vi "Process_Setting_UI.vi"(10 "ProcessSettingIn":T12[](array[typedef]), 11 "Vision_Image_In":T1(plugin-control)) -> (1 "Cancel?":bool, 2 "ProcessSettingOut":T12[](array[typedef]))   [LabVIEW 2019]
uses:
  <vilib>/vision/driver/NI_Vision_Acquisition_Software.lvlib
  <vilib>/userdefined/High Color/IMAQdx.ctl
  Controls/Process_UIAction.ctl
  Controls/UI_Process_Type.ctl
  Controls/ProcessDataEntry_Action.ctl
  Controls/Control_EnDisable_Action.ctl
  Controls/BinaryMonoParam_Type.ctl
  Controls/OperatorsParam_Type.ctl
  Controls/FiltersParam_Type.ctl
  Controls/GrayMorphologyParam_Type.ctl
  Controls/LookupTableParam.ctl
  Controls/ParticleFilterParam_Type.ctl
  Controls/MaskParam_Type.ctl
  Controls/MaskROIList_Action.ctl
  Controls/Process_Type.ctl
  <vilib>/vision/Image Controls.llb/IMAQ Image.ctl
  Controls/Process_Setting.ctl
  Controls/ExtractPlanParam_Type.ctl
  Ctrl/VisionProcessName.ctl
panel:
  out "offset past match":i32
  in  "Save":bool
  out "Vision_Image_Show":T1(plugin-control)
  in  "Tab":T2=enum."ExtractPlane"
  in  "ExtractPlanParam":T3={"Color Plane"=enum."Green"}
  in  "BinaryMonoParam":T4={"Look For"=enum."Bright Objects", "Threshold"={120.0, 255.0}} {"Threshold" scale=0.0..255.0}
  in  "OperatorsParam":T5
  out "Operators_Image":T1(plugin-control)
  in  "GrayMorphologyParam":T6={"Operation"=enum."AutoM", "Structuring Element"=[[1, 1, 1], [1, 1, 1], [1, 1, 1]], "Square/Hexa (Square)"=FALSE, "Number of iterations"=1}
  in  "FiltersParam":T7={"Kernel"=[[1.0, 1.0, 1.0], [1.0, 1.0, 1.0], [1.0, 1.0, 1.0]], "Kernel Size"=0, "Filter Size X"=0, "Filter Size Y"=0, "Tolerance %"=0, "Divider"=0.0, "FilterFunction"=enum."Smoothing - Low Pass", "Sigma"=0.0, "LThres"=0.0, "HThresh"=0.0, "Windows Size"=0} {"Kernel Size" min=3 max=7 step=2}
  in  "LookupTableParam":T8={"Function"=enum."Power X", "Power Value"=1.5}
  in  "ParticleFilterParam":T9={"Selection Values"=[], "Keep/Remove Particles (F)"=FALSE, "Reject Border? (F)"=FALSE, "Fill Holes? (F)"=FALSE, "Connectivity 4/8 (8)"=TRUE} {"Selection Values"."Measurement Parameter" items=["Center of Mass X", "Center of Mass Y", "First Pixel X", "First Pixel Y", "Bounding Rect Left", "Bounding Rect Top", "Bounding Rect Right", "Bounding Rect Bottom", "Max Feret Diameter Start X", "Max Feret Diameter Start Y", "Max Feret Diameter End X", "Max Feret Diameter End Y", "Max Horiz. Segment Length Left", "Max Horiz. Segment Length Right", "Max Horiz. Segment Length Row", "-", "Bounding Rect Width", "Bounding Rect Height", "Bounding Rect Diagonal", "Perimeter", "Convex Hull Perimeter", "Holes' Perimeter", "Max Feret Diameter", "Equivalent Ellipse Major Axis", "Equivalent Ellipse Minor Axis", "Equivalent Ellipse Minor Axis (Feret)", "Equivalent Rect Long Side", "Equivalent Rect Short Side", "Equivalent Rect Diagonal", "Equivalent Rect Short Side (Feret)", "Average Horiz. Segment Length", "Average Vert. Segment Length", "Hydraulic Radius", "Waddel Disk Diameter", "-", "Area", "Holes' Area", "Particle & Holes' Area", "Convex Hull Area", "Image Area", "-", "Number of Holes", "Number of Horiz. Segments", "Number of Vert. Segments", "-", "Orientation", "Max Feret Diameter Orientation", "-", "% Area/Image Area", "% Area/(Particle & Holes' Area)", "Ratio of Equivalent Ellipse Axes", "Ratio of Equivalent Rect Sides", "-", "Elongation Factor", "Compactness Factor", "Heywood Circularity Factor", "Type Factor", "-", "Sum X", "Sum Y", "Sum XX", "Sum XY", "Sum YY", "Sum XXX", "Sum XXY", "Sum XYY", "Sum YYY", "-", "Moment of Inertia XX", "Moment of Inertia XY", "Moment of Inertia YY", "Moment of Inertia XXX", "Moment of Inertia XXY", "Moment of Inertia XYY", "Moment of Inertia YYY", "Norm. Moment of Inertia XX", "Norm. Moment of Inertia XY", "Norm. Moment of Inertia YY", "Norm. Moment of Inertia XXX", "Norm. Moment of Inertia XXY", "Norm. Moment of Inertia XYY", "Norm. Moment of Inertia YYY", "Hu Moment 1", "Hu Moment 2", "Hu Moment 3", "Hu Moment 4", "Hu Moment 5", "Hu Moment 6", "Hu Moment 7"]; "Selection Values"."Range Lower Value" format="%.2f"; "Selection Values"."Range Upper Value" format="%.2f"}
  in  "MaskParam":T11
  in  "Remove":bool
  in  "Add":bool
  in  "Process Steps":i32(listbox)
  in  "Cancel":bool
  in  "Done":bool
  # "Minimum"
  # "Maximum"
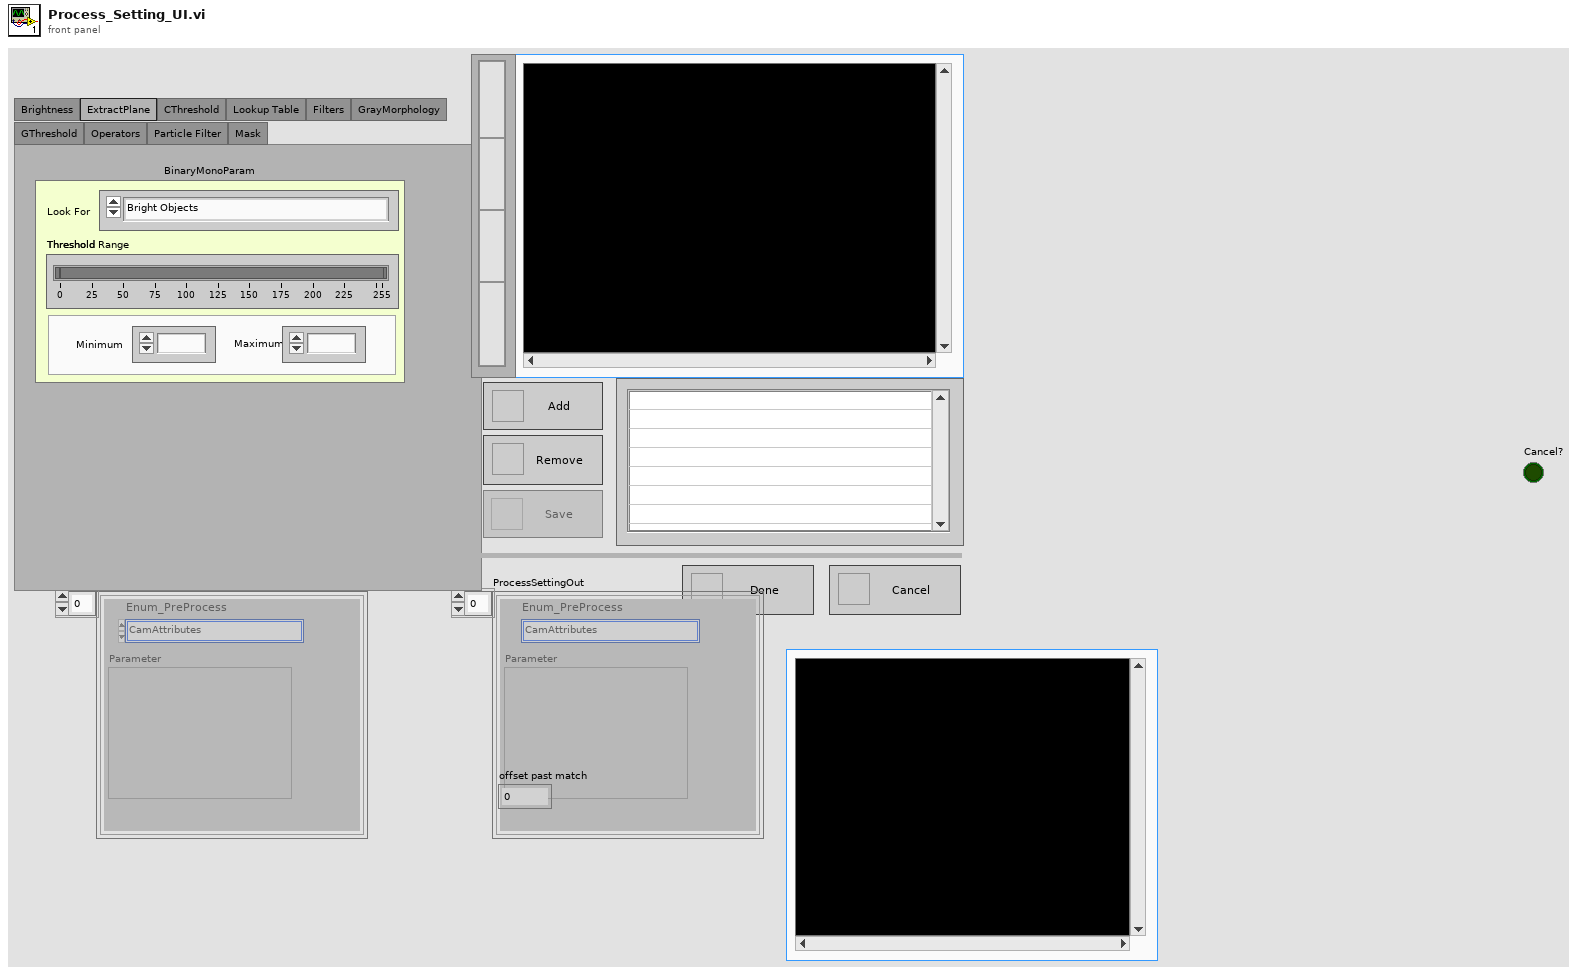
[diagram p1: front panel]
types:
  T1 = typedef "IMAQ Image.ctl" = refnum<image>
  T2 = typedef "UI_Process_Type.ctl" = enum32{"None", "Brightness", "ExtractPlane", "CThreshold", "Lookup Table", "Filters", "GrayMorphology", "GThreshold", "Operators", "Particle Filter", "Mask"}
  T3 = typedef "ExtractPlanParam_Type.ctl" = cluster{"Color Plane":enum16{"Red", "Green", "Blue", "Hue", "Saturation", "Luminance", "Value", "Intensity"}}
  T4 = typedef "BinaryMonoParam_Type.ctl" = cluster{"Look For":enum16{"Bright Objects", "Dark Objects", "Gray Objects"}, "Threshold":cluster{dbl, dbl}}
  T5 = typedef "OperatorsParam_Type.ctl" = cluster{"Actions":enum16{"Add", "Subtract", "Multiply", "Divide", "Multiply Divide", "Modulo", "Absolutio Difference", "---------------------------------", "And", "Not And", "Or", "Not Or", "Exclusive Or", "Not Exclusive Or", "Logical Difference", "----------------------------------", "Mask"}, "Select Mode:":enum32{"Constant", "Image"}, "Color Box":u32, "Image Path":path}
  T6 = typedef "GrayMorphologyParam_Type.ctl" = cluster{"Operation":enum32{"AutoM", "Close", "Dilate", "Erode", "Gradient", "Gradient in", "Gradient out", "HitMiss", "Open", "PClose", "POpen", "Thick", "Thin"}, "Structuring Element":i32[][], "Square/Hexa (Square)":bool, "Number of iterations":i32}
  T7 = typedef "FiltersParam_Type.ctl" = cluster{"Kernel":sgl[][], "Kernel Size":i32, "Filter Size X":i32, "Filter Size Y":i32, "Tolerance %":i32, "Divider":sgl, "FilterFunction":enum16{"Smoothing - Low Pass", "Smoothing - Local Average", "Smoothing - Guassian", "Smoothing - Median", "------------------------------------", "Edge Detection - Laplacian", "Edge Detection - Diff", "Edge Detection - Prewitt", "Edge Detection - Sobel", "Edge Detection - Roberts", "Edge Detection - Canny", "Edge Detection - Gradient", "Edge Detection - Sigma", "----------------------------------------", "Convolution - Highlight Details", "Convolution - Custom"}, "Sigma":sgl, "LThres":sgl, "HThresh":sgl, "Windows Size":i32}
  T8 = typedef "LookupTableParam.ctl" = cluster{"Function":enum16{"Equalizer", "Reverse", "Logarithmic", "Exponential", "Square", "Square Root", "Power X", "Power 1/X"}, "Power Value":sgl}
  T9 = typedef "ParticleFilterParam_Type.ctl" = cluster{"Selection Values":cluster{"Measurement Parameter":T10, "Range Lower Value":dbl, "Range Upper Value":dbl, "Range":bool, "Measurement Type":bool}[], "Keep/Remove Particles (F)":bool, "Reject Border? (F)":bool, "Fill Holes? (F)":bool, "Connectivity 4/8 (8)":bool}
  T10 = typedef "Particle Parameters" = i32
  T11 = typedef "MaskParam_Type.ctl" = cluster{"Function":enum16{"Inside", "Outside"}, "ROI List":i32, "ROI":cluster{"Global Rectangle":i32[], "Contours":cluster{"Contour Type":u32, "ROI Type":u32, "Points":i32[]}[]}[], "Creat ROI":bool, "Delete ROI":bool, "Enabled/Disabled":bool, "Color Box":u32, "Last Mouse Position":cluster{"X":i32, "Y":i32}}
  T12 = typedef "Process_Setting.ctl" = cluster{"Enum_PreProcess":T13, "Parameter":string}
  T13 = typedef "VisionProcessName.ctl" = enum16{"*CamParameter*", "CamAttributes", "*Preprocess*", "CG_Brightness", "C_Plane Extraction", "C_Threshold", "G_Lookup Table", "G_Threshold"}
  T14 = enum8{"Enabled", "Disabled", "Disabled and Grayed Out"}
  T15 = typedef "ProcessDataEntry_Action.ctl" = enum16{"Intial", "UpdateSteps", "ReallAllSteps", "ReadStep"}
  T16 = typedef "Image Type" = u32
  T17 = typedef "Process_UIAction.ctl" = cluster{"Process_UIActionCmd":enum16{"Init", "SingleStep", "RunAllSteps", "RemoveSteps", "PreTest", "Exist"}, "Process_UIParam":variant, "EventName":string}
  T18 = typedef "IMAQdx.ctl" = refnum<k21>
  T19 = typedef "Control_EnDisable_Action.ctl" = enum16{"Store Ref", "Add Mode", "Select Mode", "Enable All", "OnePageEnable", "OnePageDisable", "AllPageDisable", "AllPageEnable", "PageRefOut"}
  T20 = cluster{"Color Plane":enum16{"Red", "Green", "Blue", "Hue", "Saturation", "Luminance", "Value", "Intensity"}}
  T21 = typedef "MaskROIList_Action.ctl" = enum16{"initialize", "SaveAll", "ReadAll", "Append", "Replace", "DeleteIndex"}
  T22 = typedef "Process_Type.ctl" = enum16{"None", "ExtractPlane", "BinaryMono", "Operators", "GrayMorphology", "Filters", "Lookup Table", "Particle Filter", "Mask"}
  T23 = enum16{"Smoothing - Low Pass", "Smoothing - Local Average", "Smoothing - Guassian", "Smoothing - Median", "------------------------------------", "Edge Detection - Laplacian", "Edge Detection - Diff", "Edge Detection - Prewitt", "Edge Detection - Sobel", "Edge Detection - Roberts", "Edge Detection - Canny", "Edge Detection - Gradient", "Edge Detection - Sigma", "----------------------------------------", "Convolution - Highlight Details", "Convolution - Custom"}
  T24 = enum16{"Bright Objects", "Dark Objects", "Gray Objects"}
  T25 = cluster{"Look For":enum16{"Bright Objects", "Dark Objects", "Gray Objects"}, "Threshold Range Gray":cluster{dbl, dbl}}
  T26 = cluster{"Global Rectangle":i32[], "Contours":cluster{"Contour Type":u32, "ROI Type":u32, "Points":i32[]}[]}
  T27 = cluster{"Contour Type":u32, "ROI Type":u32, "Points":i32[]}[]
  T28 = cluster{"Global Rectangle":i32[], "Contours":cluster{"Contour Type":u32, "ROI Type":u32, "Points":i32[]}[]}[]
  T29 = typedef "UI_Process_Type.ctl" = enum32{"None", "Brightness", "ExtractPlane", "Lookup Table", "Filters", "GrayMorphology", "BinaryMono", "Operators", "Particle Filter", "Mask"}
  T30 = enum16{"Init", "SingleStep", "RunAllSteps", "RemoveSteps", "PreTest", "Exist"}
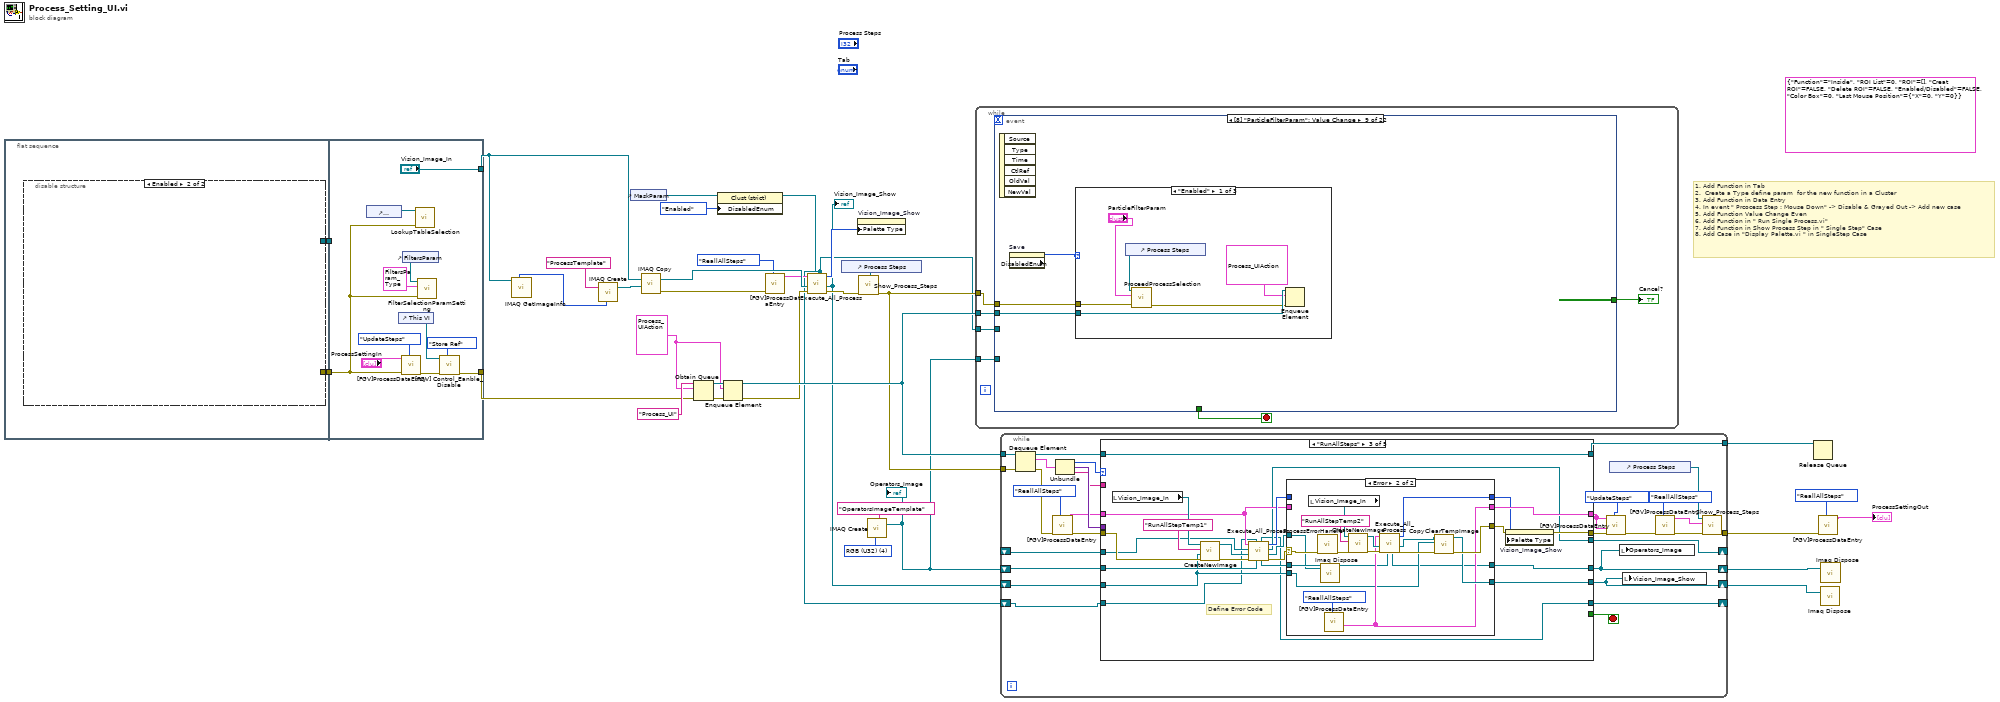
[diagram p0: block diagram]
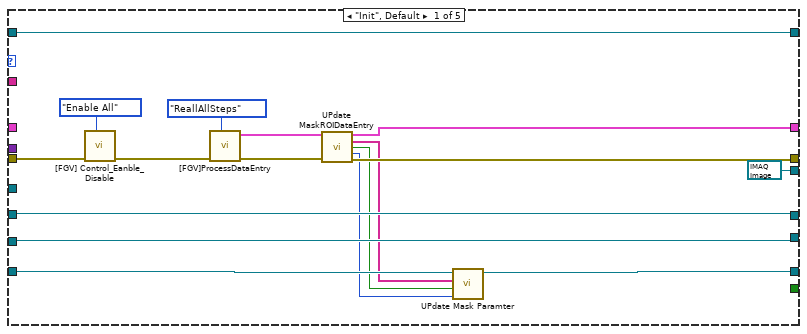
[diagram p2: hidden frame]
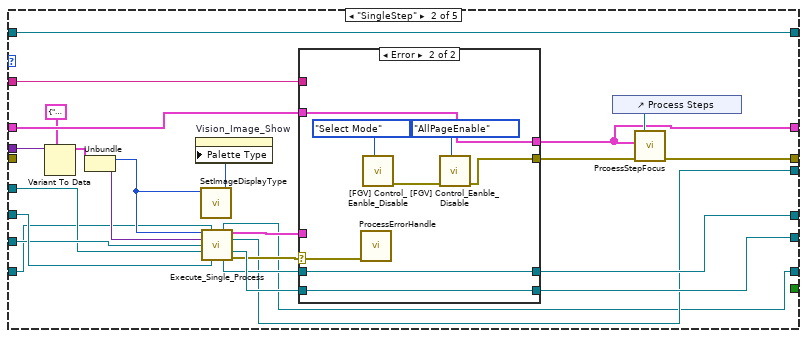
[diagram p3: hidden frame]
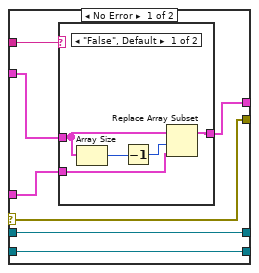
[diagram p4: hidden frame]
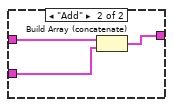
[diagram p5: hidden frame]
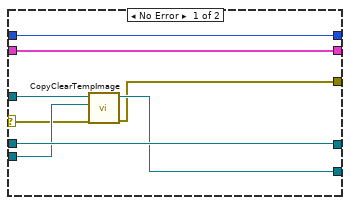
[diagram p6: hidden frame]
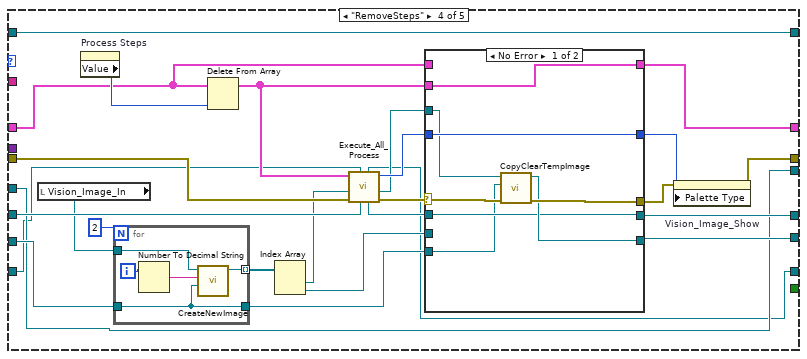
[diagram p7: hidden frame]
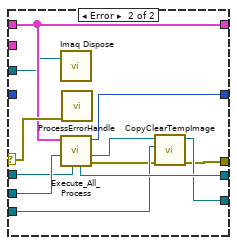
[diagram p8: hidden frame]
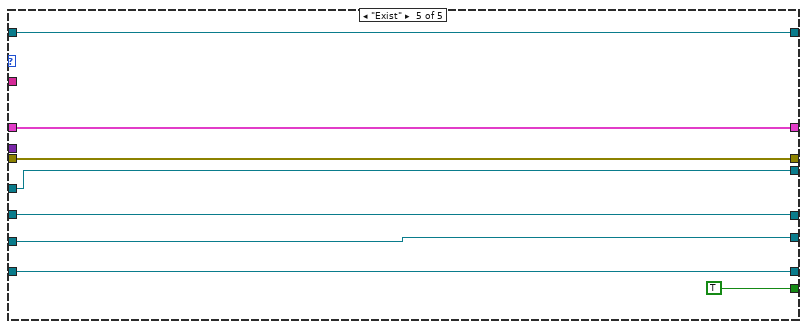
[diagram p9: hidden frame]
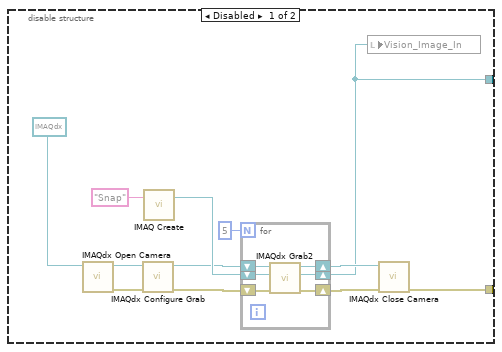
[diagram p10: hidden frame]
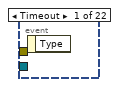
[diagram p11: hidden frame]
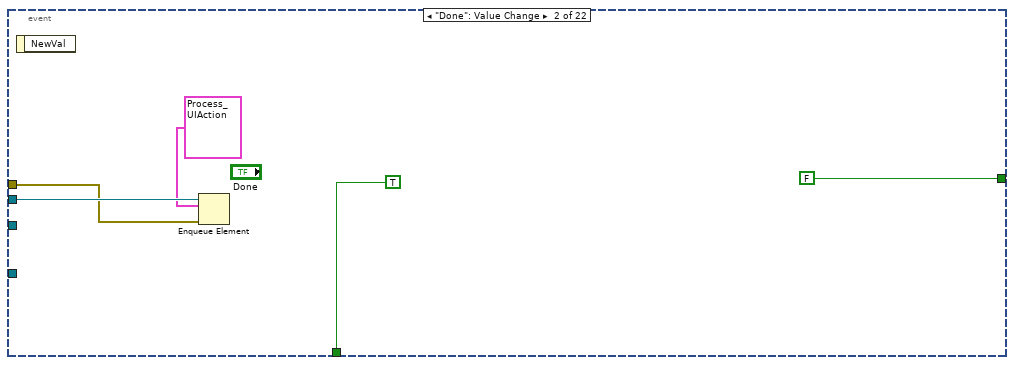
[diagram p12: hidden frame]
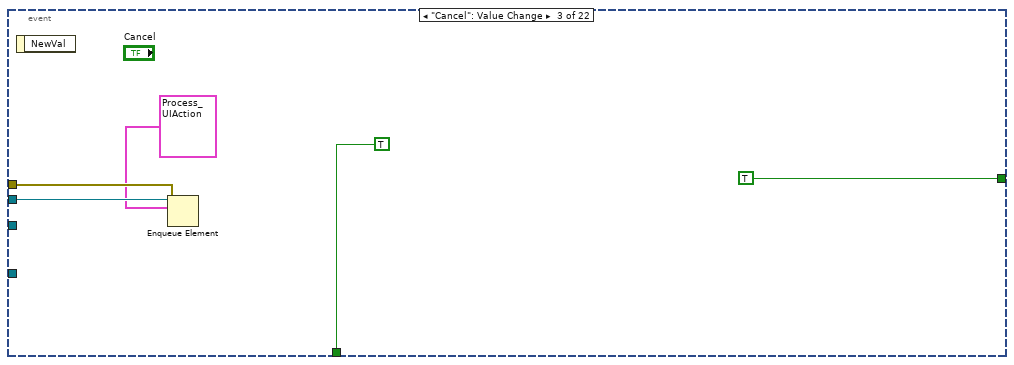
[diagram p13: hidden frame]
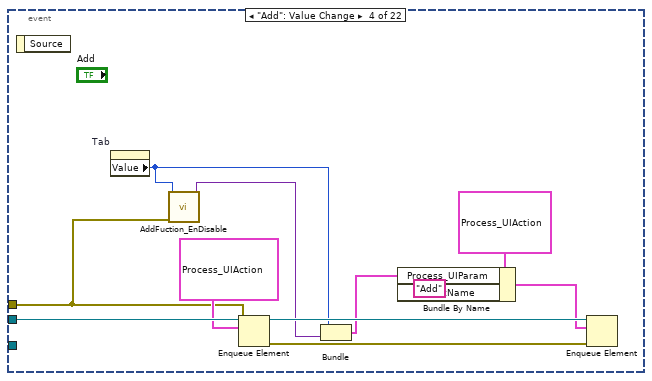
[diagram p14: hidden frame]
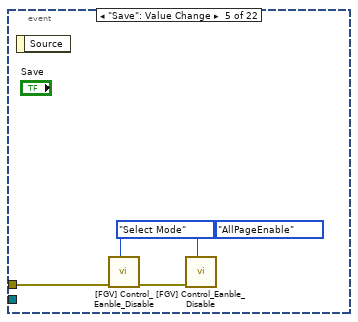
[diagram p15: hidden frame]
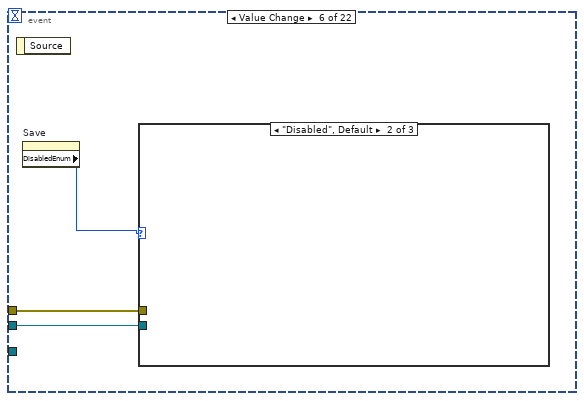
[diagram p16: hidden frame]
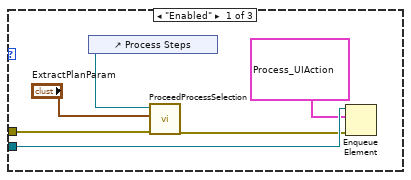
[diagram p17: hidden frame]
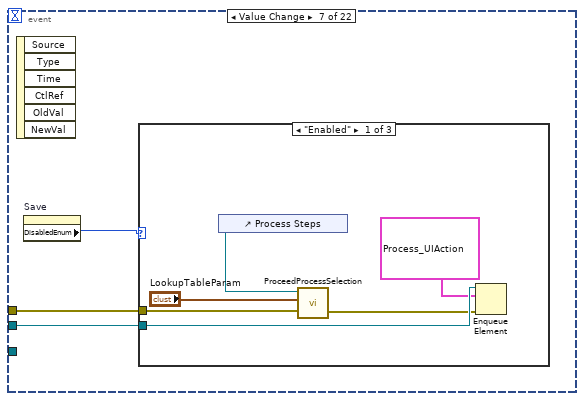
[diagram p19: hidden frame]
diagram:
  (unwired) T11 {"Function"=enum."Inside", "ROI List"=0, "ROI"=[], "Creat ROI"=FALSE, "Delete ROI"=FALSE, "Enabled/Disabled"=FALSE, "Color Box"=0, "Last Mouse Position"={"X"=0, "Y"=0}} ("MaskParam")
  w18 = T16 4 items=["Grayscale (U8)", "Grayscale (I16)", "Grayscale (SGL)", "Complex (CSG)", "RGB (U32)", "HSL (U32)", "RGB (U64)", "Grayscale (U16)"] ("Image Type")
  w21 = T17 {"Process_UIActionCmd"=enum."Init", "Process_UIParam"=variant, "EventName"=""} ("Process_UIAction")
  # "1. Add Function in Tab \n2.  Create a Type define param  for the new function in a Cluster \n3. Add Function in Data Entry\n4. In event \" Prcocess Step : Mouse Down\" -> Disable & Grayed Out -> Add new case \n5. Add Function Value Change Even\n6. Add Function in \" Run Single Process.vi\"\n7. Add Function in Show Process Step in \" Single Step\" Case\n8. Add Case in \"Display Palette.vi \" in SingleStep Case"
  n1 = flat-sequence {
    tunnel: [w37] -> w31
    tunnel: [w36] -> w30
    tunnel: ["Vision_Image_In"] -> w33
    tunnel: [w62] -> w14
    tunnel: w31 -> [w57]
    tunnel: w30 -> [_]
    frame #0 {
      n2 = disable-structure shown="Enabled" {
        disable-tunnel: [w43 _] -> w37
        disable-tunnel: [w38 _] -> w36
        frame Disabled {
          n3 = call <vilib>:"IMAQdx Open Camera.vi"("Session In"=T18 refnum) -> ("error out"=w41:errorcluster, "Session Out"=w48:T18)  [unwired: 2 in, 7 out]
          n4 = call <vilib>:"IMAQdx Configure Grab.vi"("error in"=w41, "Session In"=w48) -> ("error out"=w40:errorcluster, "Session Out"=w42:T18)  [unwired: 8 in]
          n5 = call "IMAQ Create"("Image Name"="Snap") -> ("New Image"=w46:T1)  [unwired: 3 in, 2 out]
          n6 = for {
            N: 5 -> [_]
            shift-right: [w52] -> w38
            shift-left: w46 -> [w53]
            shift-right: [w55] -> w49
            shift-left: w42 -> [w51]
            shift-right: [w54] -> w47
            shift-left: w40 -> [w50]
            n7 = call <vilib>:"IMAQdx Grab2.vi"("error in"=w50, "Image In"=w53, "Session In"=w51) -> ("error out"=w54:errorcluster, "Image Out"=w52:T1, "Session Out"=w55:T18)  [unwired: 5 in, 1 out]
          }
          n8 = local write "Vision_Image_In"(w38) -> ()
          n9 = call <vilib>:"IMAQdx Close Camera.vi"("error in"=w47, "Session In"=w49) -> ("error out"=w43:errorcluster)  [unwired: 9 out]
        }
        frame Enabled {
        }
      }
    }
    frame #1 {
      n10 = control-ref of="LookupTableParam"() -> (w56:refnum<vi>)
      n11 = control-ref of="This VI"() -> (w61:refnum<vi>)
      n12 = call "[FGV]ProcessDataEntry.vi"("ProcessDataEntry_Action"=ProcessDataEntry_Action."UpdateSteps", "Error In"=w57, "AllProcessSetting In"="ProcessSettingIn") -> ("Error Out"=w63:errorcluster)  [unwired: 5 in, 3 out]
      n13 = control-ref of="FiltersParam"() -> (w59:refnum<vi>)
      n14 = call "LookupTableSelection.vi"("Error In"=w57, "LookupTableParam"=w56) -> ()  [unwired: 9 in, 1 out]
      n15 = call "FilterSelectionParamSetting.vi"("Error In"=w57, 10:"FiltersParam"=T7 {"Kernel"=[[1.0, 1.0, 1.0], [1.0, 1.0, 1.0], [1.0, 1.0, 1.0]], "Kernel Size"=0, "Filter Size X"=0, "Filter Size Y"=0, "Tolerance %"=0, "Divider"=0.0, "FilterFunction"=enum."Smoothing - Low Pass", "Sigma"=0.0, "LThres"=0.0, "HThresh"=0.0, "Windows Size"=0} ("FiltersParam"), 11:"FiltersParam"=w59) -> ()  [unwired: 8 in, 1 out]
      n16 = call "[FGV] Control_Eanble_Disable.vi"("Control_EnDisable_Action"=Control_EnDisable_Action."Store Ref", "Error In"=w63, "This VI"=w61) -> ("Error Out"=w62:errorcluster)  [unwired: 7 in, 1 out]
    }
  }
  n17 = call "IMAQ GetImageInfo"("Image"=w33) -> ("Image Type"=w19:T16)  [unwired: 3 in, 7 out]
  n18 = call "IMAQ Create"("Image Name"="ProcessTemplate", "Image Type"=w19) -> ("New Image"=w34:T1)  [unwired: 3 in, 1 out]
  n19 = control-ref of="MaskParam"() -> (w4:refnum<vi>)
  n20 = call "IMAQ Copy"("Image Dst"=w34, "Image Src"=w33) -> ("error out"=w10:errorcluster, "Image Dst Out"=w29:T1)  [unwired: 4 in]
  n21 = Obtain Queue(name (unnamed)="Process_UI", element data type=w21, error in (no error)=w14) -> (queue out=w26:refnum<queue>, error out=w22:errorcluster)  [unwired: 2 in, 1 out]
  n22 = property class="Clust (strict)"(reference=w4, "DisabledEnum"=T14."Enabled" ("Disabled")) -> (reference out=w2:refnum<vi>)  [unwired: 1 in, 1 out]
  n23 = Enqueue Element(queue=w26, element=w21, error in (no error)=w22) -> (queue out=w23:refnum<queue>, error out=w5:errorcluster)  [unwired: 1 in, 1 out]
  n24 = call "[FGV]ProcessDataEntry.vi"("ProcessDataEntry_Action"=ProcessDataEntry_Action."ReallAllSteps", "Error In"=w10) -> ("AllProcessSettingOut"=w9:T12[])  [unwired: 6 in, 3 out]
  n25 = call "Execute_All_Process.vi"("MaskParam 2"=w2, "error in (no error)"=w5, "ImageIn"=w29, "ProcessSettingIn"=w9) -> ("error out"=w16:errorcluster, "Image Out"=w15:T1, "Palette Type"=w28:u32, "MaskParam 3"=w3:refnum<vi>)  [unwired: 2 in, 2 out]
  "Vision_Image_Show" <- w15
  n26 = control-ref of="Process Steps"() -> (w32:refnum<vi>)
  n27 = property on="Vision_Image_Show" class="ImageControl"("Palette Type"=w28) -> ()  [unwired: 2 in, 2 out]
  n28 = call "Show_Process_Steps.vi"("error in (no error)"=w16, "ProcessSteps"=w32) -> ("error out"=w17:errorcluster)  [unwired: 9 in]
  n29 = call "IMAQ Create"("Image Name"="OperatorsImageTemplate", "Image Type"=w18) -> ("New Image"=w12:T1)  [unwired: 3 in, 1 out]
  "Operators_Image" <- w12
  n30 = while {
    tunnel: w17 -> [w70]
    tunnel: w23 -> [w71]
    tunnel: w12 -> [w69]
    tunnel: w3 -> [w67]
    stop <- w72 stop-if-true
    n31 = event shown="[8] \"ParticleFilterParam\": Value Change" {
      selector: _ -> [_ _ _ _ _ _ _ _ _ _ _ _ _ _ _ _ _ _ _ _ _ _]
      dyn-events: _ -> [_ _ _ _ _ _ _ _ _ _ _ _ _ _ _ _ _ _ _ _ _ _]
      timeout: _ -> [_ _ _ _ _ _ _ _ _ _ _ _ _ _ _ _ _ _ _ _ _ _]
      tunnel: [_ TRUE TRUE _ _ _ _ _ _ _ _ _ _ _ _ _ _ _ _ _ _ _] -> w72
      tunnel: w71 -> [_ w76 w81 w93 _ w100 w109 w118 w127 w143 _ _ w170 w189 _ w232 w237 w274 w310 w322 w348 w385]
      tunnel: w70 -> [_ w75 w80 w87 w94 w98 w107 w116 w125 w142 w149 w150 w171 w183 _ w231 w236 _ w311 w320 w349 _]
      tunnel: w69 -> [_ _ _ _ _ _ _ _ _ _ _ _ w169 _ _ _ _ _ _ _ w346 _]
      tunnel: [_ FALSE ("Cancel?") TRUE ("Cancel?") _ _ _ _ _ _ _ _ _ _ _ _ _ _ _ _ _ _ _] -> w68
      tunnel: w67 -> [_ _ _ _ _ _ _ _ _ _ _ _ _ _ _ _ w234 w272 w312 w321 w347 w378]
      event Timeout {
        n32 = event-data() -> ()  [unwired: 1 in, 1 out]
      }
      event "Done": Value Change {
        n33 = event-data() -> ()  [unwired: 1 in, 1 out]
        n34 = Enqueue Element(queue=w76, element=T17 {"Process_UIActionCmd"=enum."Exist", "Process_UIParam"=variant, "EventName"=""}, error in (no error)=w75) -> ()  [unwired: 1 in, 3 out]
      }
      event "Cancel": Value Change {
        n35 = event-data() -> ()  [unwired: 1 in, 1 out]
        n36 = Enqueue Element(queue=w81, element=T17 {"Process_UIActionCmd"=enum."Exist", "Process_UIParam"=variant, "EventName"=""}, error in (no error)=w80) -> ()  [unwired: 1 in, 3 out]
      }
      event "Add": Value Change {
        n37 = event-data() -> ()  [unwired: 1 in, 1 out]
        n38 = property on="Tab" class="TabCtl (strict)"() -> ("Value"=w86:T2)  [unwired: 2 in, 2 out]
        n39 = call "AddFuction_EnDisable.vi"("error in (no error)"=w87, "Value"=w86) -> ("Selected Param"=w84:variant)  [unwired: 9 in]
        n40 = Enqueue Element(queue=w93, element=T17 {"Process_UIActionCmd"=enum."RunAllSteps", "Process_UIParam"=variant, "EventName"=""}, error in (no error)=w87) -> (queue out=w91:refnum<queue>, error out=w83:errorcluster)  [unwired: 1 in, 1 out]
        n41 = Bundle("Value"=w86, "Selected Param"=w84) -> (w89:cluster{"Value":T2, "Selected Param":variant})  [unwired: 1 in]
        n42 = Bundle By Name(cluster=T17 {"Process_UIActionCmd"=enum."SingleStep", "Process_UIParam"=variant, "EventName"=""} ("element"), "Process_UIParam"=w89, "EventName"="Add") -> (w88:T17)
        n43 = Enqueue Element(queue=w91, element=w88, error in (no error)=w83) -> ()  [unwired: 1 in, 3 out]
      }
      event "Save": Value Change {
        n44 = event-data() -> ()  [unwired: 1 in, 1 out]
        n45 = call "[FGV] Control_Eanble_Disable.vi"("Control_EnDisable_Action"=Control_EnDisable_Action."Select Mode", "Error In"=w94) -> ("Error Out"=w96:errorcluster)  [unwired: 8 in, 1 out]
        n46 = call "[FGV] Control_Eanble_Disable.vi"("Control_EnDisable_Action"=Control_EnDisable_Action."AllPageEnable", "Error In"=w96) -> ()  [unwired: 8 in, 2 out]
      }
      event Value Change {
        n47 = event-data() -> ()  [unwired: 1 in, 1 out]
        n48 = property on="Save" class="Bool"() -> ("DisabledEnum"=w99:T14)  [unwired: 2 in, 2 out]
        n49 = case shown="\"Disabled\", Default" w99 {
          tunnel: w100 -> [w106 _ _]
          tunnel: w98 -> [w101 _ _]
          frame "Enabled" {
            n50 = control-ref of="Process Steps"() -> (w103:refnum<vi>)
            n51 = call "ProceedProcessSelection.vi"("Error In"=w101, "Selected Param"="ExtractPlanParam", "MulticolumnListbox in"=w103) -> ("error out"=w104:errorcluster)  [unwired: 8 in]
            n52 = Enqueue Element(queue=w106, element=T17 {"Process_UIActionCmd"=enum."RunAllSteps", "Process_UIParam"=variant, "EventName"=""}, error in (no error)=w104) -> ()  [unwired: 1 in, 3 out]
          }
          frame "Disabled", Default {
          }
          frame "Disabled and Grayed Out" {
          }
        }
      }
      event Value Change {
        n53 = event-data() -> ()  [unwired: 1 in, 6 out]
        n54 = property on="Save" class="Bool"() -> ("DisabledEnum"=w108:T14)  [unwired: 2 in, 2 out]
        n55 = case shown="\"Enabled\"" w108 {
          tunnel: w109 -> [w115 _ _]
          tunnel: w107 -> [w111 _ _]
          frame "Enabled" {
            n56 = control-ref of="Process Steps"() -> (w112:refnum<vi>)
            n57 = call "ProceedProcessSelection.vi"("Error In"=w111, "Selected Param"="LookupTableParam", "MulticolumnListbox in"=w112) -> ("error out"=w113:errorcluster)  [unwired: 8 in]
            n58 = Enqueue Element(queue=w115, element=T17 {"Process_UIActionCmd"=enum."RunAllSteps", "Process_UIParam"=variant, "EventName"=""}, error in (no error)=w113) -> ()  [unwired: 1 in, 3 out]
          }
          frame "Disabled", Default {
          }
          frame "Disabled and Grayed Out" {
          }
        }
      }
      event Value Change {
        n59 = event-data() -> ()  [unwired: 1 in, 1 out]
        n60 = property on="Save" class="Bool"() -> ("DisabledEnum"=w117:T14)  [unwired: 2 in, 2 out]
        n61 = case shown="\"Enabled\"" w117 {
          tunnel: w118 -> [w124 _ _]
          tunnel: w116 -> [w120 _ _]
          frame "Enabled" {
            n62 = control-ref of="Process Steps"() -> (w121:refnum<vi>)
            n63 = call "ProceedProcessSelection.vi"("Error In"=w120, "Selected Param"="GrayMorphologyParam", "MulticolumnListbox in"=w121) -> ("error out"=w122:errorcluster)  [unwired: 8 in]
            n64 = Enqueue Element(queue=w124, element=T17 {"Process_UIActionCmd"=enum."RunAllSteps", "Process_UIParam"=variant, "EventName"=""}, error in (no error)=w122) -> ()  [unwired: 1 in, 3 out]
          }
          frame "Disabled", Default {
          }
          frame "Disabled and Grayed Out" {
          }
        }
      }
      event Value Change {
        n65 = event-data() -> ()  [unwired: 1 in, 6 out]
        n66 = property on="Save" class="Bool"() -> ("DisabledEnum"=w126:T14)  [unwired: 2 in, 2 out]
        n67 = case shown="\"Enabled\"" w126 {
          tunnel: w127 -> [w133 _ _]
          tunnel: w125 -> [w129 _ _]
          frame "Enabled" {
            n68 = control-ref of="Process Steps"() -> (w130:refnum<vi>)
            n69 = call "ProceedProcessSelection.vi"("Error In"=w129, "Selected Param"="ParticleFilterParam", "MulticolumnListbox in"=w130) -> ("error out"=w131:errorcluster)  [unwired: 8 in]
            n70 = Enqueue Element(queue=w133, element=T17 {"Process_UIActionCmd"=enum."RunAllSteps", "Process_UIParam"=variant, "EventName"=""}, error in (no error)=w131) -> ()  [unwired: 1 in, 3 out]
          }
          frame "Disabled", Default {
          }
          frame "Disabled and Grayed Out" {
          }
        }
      }
      event Value Change {
        n71 = event-data() -> ()  [unwired: 1 in, 6 out]
        n72 = property on="Save" class="Bool" props=["DisabledEnum"]() -> ()  [unwired: 2 in, 3 out]
        n73 = control-ref of="FiltersParam"() -> (w136:refnum<vi>)
        n74 = call "FilterSelectionParamSetting.vi"("Error In"=w142, 10:"FiltersParam"="FiltersParam", 11:"FiltersParam"=w136) -> ("Error Out"=w137:errorcluster)  [unwired: 8 in]
        n75 = call "FilterParamInitial.vi"("Error In"=w137, "FiltersParam"=w136) -> ("Error Out"=w138:errorcluster, "FiltersParam Out"=w134:T7)  [unwired: 8 in]
        n76 = control-ref of="Process Steps"() -> (w140:refnum<vi>)
        n77 = call "ProceedProcessSelection.vi"("Error In"=w138, "Selected Param"=w134, "MulticolumnListbox in"=w140) -> ("error out"=w139:errorcluster)  [unwired: 8 in]
        n78 = Enqueue Element(queue=w143, element=T17 {"Process_UIActionCmd"=enum."RunAllSteps", "Process_UIParam"=variant, "EventName"=""}, error in (no error)=w139) -> ()  [unwired: 1 in, 3 out]
      }
      event Value Change {
        w147 = T7 {"Kernel"=[[1.0, 1.0, 1.0], [1.0, 1.0, 1.0], [1.0, 1.0, 1.0]], "Kernel Size"=3, "Filter Size X"=0, "Filter Size Y"=0, "Tolerance %"=0, "Divider"=0.0, "FilterFunction"=enum."Smoothing - Low Pass", "Sigma"=0.0, "LThres"=0.0, "HThresh"=0.0, "Windows Size"=0}  # FiltersParam
        n79 = event-data() -> ("NewVal"=w146:T23)  [unwired: 1 in, 5 out]
        n80 = control-ref of="FiltersParam"() -> (w144:refnum<vi>)
        n81 = Bundle By Name(cluster=w147, "FilterFunction"=w146) -> (w145:T7)
        n82 = call "FilterParamInitial.vi"("Error In"=w149, "FiltersParam"=w144) -> ("Error Out"=w148:errorcluster)  [unwired: 8 in, 1 out]
        n83 = call "FilterSelectionParamSetting.vi"("Error In"=w148, 10:"FiltersParam"=w145, 11:"FiltersParam"=w144) -> ()  [unwired: 8 in, 1 out]
      }
      event Value Change {
        n84 = event-data() -> ()  [unwired: 1 in, 6 out]
        n85 = control-ref of="LookupTableParam"() -> (w151:refnum<vi>)
        n86 = call "LookupTableSelection.vi"("Error In"=w150, "LookupTableParam"=w151) -> ()  [unwired: 9 in, 1 out]
      }
      event Value Change {
        w154 = 3 ("y")
        n87 = event-data() -> ("NewVal.Select Mode:"=w164:enum32{"Constant", "Image"}, "NewVal.Image Path"=w157:path)  [unwired: 1 in]
        n88 = Path To String(path=w157) -> (string=w156:string)
        n89 = String Length(string=w156) -> (length=w155:i32)
        n90 = Subtract(x=w155, y=w154) -> (x-y=w152:i32)
        n91 = String Subset(string=w156, offset (0)=w152, length (rest)=w154) -> (substring=w153:string)
        n92 = Equal?(x=enum32{"Constant", "Image"}."Image", y=w164) -> (x = y?=w162:bool)
        n93 = Not Equal?(x=w157, y=path "") -> (x != y?=w160:bool)
        n94 = Search 1D Array(1D array=string[] ["png", "jpg", "bmp"], element=w153) -> (index of element=w166:i32)  [unwired: 1 in]
        n95 = Equal?(x=-1, y=w166) -> (x = y?=w159:bool)
        n96 = Compound Arithmetic op=AND(w162, w160, w159) -> (w158:bool)
        n97 = property on="Save" class="Bool"() -> ("DisabledEnum"=w168:T14)  [unwired: 2 in, 2 out]
        n98 = case shown="True" w158 {
          frame False {
          }
          frame True {
            n99 = One Button Dialog(message="Input File Type Error", button name ("OK")="OK") -> ()  [unwired: 1 out]
            n100 = property on="Image Path" class="Path"("Value"=path "") -> ()  [unwired: 2 in, 2 out]
          }
        }
        n101 = case shown="\"Enabled\"" w168 {
          tunnel: w171 -> [w178 _ _]
          tunnel: w170 -> [w176 _ _]
          tunnel: w169 -> [_ _ _]
          frame "Enabled" {
            n102 = control-ref of="Process Steps"() -> (w180:refnum<vi>)
            n103 = call "ProceedProcessSelection.vi"("Error In"=w178, "Selected Param"="OperatorsParam", "MulticolumnListbox in"=w180) -> ("error out"=w177:errorcluster)  [unwired: 8 in]
            n104 = Enqueue Element(queue=w176, element=T17 {"Process_UIActionCmd"=enum."RunAllSteps", "Process_UIParam"=variant, "EventName"=""}, error in (no error)=w177) -> ()  [unwired: 1 in, 3 out]
          }
          frame "Disabled", Default {
          }
          frame "Disabled and Grayed Out" {
          }
        }
      }
      event Mouse Up {
        n105 = event-data() -> ()  [unwired: 1 in, 1 out]
        n106 = control-ref of="BinaryMonoParam"() -> (w185:refnum<vi>)
        n107 = Unbundle("BinaryMonoParam") -> ("Look For"=w186:T24, "Threshold"=w187:cluster{dbl, dbl})
        n108 = property on="Save" class="Bool"() -> ("DisabledEnum"=w188:T14)  [unwired: 2 in, 2 out]
        n109 = call "BinaryMono_SliderControl.vi"("NewVal"="BinaryMonoParam", "Error In"=w183, "Look For"=w186, "Threshold Range Gray"=w187, "Cluster in"=w185) -> ("Error Out"=w182:errorcluster, "BinaryMonoParam Out"=w181:T25)  [unwired: 5 in]
        n110 = case shown="\"Enabled\"" w188 {
          tunnel: w189 -> [w195 _ _]
          tunnel: w182 -> [w191 _ _]
          tunnel: w181 -> [w190 _ _]
          frame "Enabled" {
            n111 = control-ref of="Process Steps"() -> (w194:refnum<vi>)
            n112 = call "ProceedProcessSelection.vi"("Error In"=w191, "Selected Param"=w190, "MulticolumnListbox in"=w194) -> ("error out"=w192:errorcluster)  [unwired: 8 in]
            n113 = Enqueue Element(queue=w195, element=T17 {"Process_UIActionCmd"=enum."RunAllSteps", "Process_UIParam"=variant, "EventName"=""}, error in (no error)=w192) -> ()  [unwired: 1 in, 3 out]
          }
          frame "Disabled", Default {
          }
          frame "Disabled and Grayed Out" {
          }
        }
      }
      event "Process Steps": Mouse Down {
        n114 = event-data() -> ("Mods.Double Click"=w197:bool)  [unwired: 1 in]
        n115 = property on="Save" class="Bool"() -> ("DisabledEnum"=w196:T14)  [unwired: 2 in, 2 out]
        n116 = case shown="\"Disabled and Grayed Out\"" w196 {
          tunnel: w197 -> [_ _ w198]
          frame "Enabled" {
          }
          frame "Disabled", Default {
          }
          frame "Disabled and Grayed Out" {
            n117 = case shown="True" w198 {
              frame False {
              }
              frame True {
                n118 = property on="Process Steps" class="MCListbox (strict)"() -> ("Value"=w202:i32)  [unwired: 2 in, 2 out]
                n119 = call "[FGV]ProcessDataEntry.vi"("ProcessDataEntry_Action"=ProcessDataEntry_Action."ReadStep", "Prcocess Step"=w202) -> ("ProcessSetting Out"=w201:T12)  [unwired: 6 in, 3 out]
                n120 = Unbundle By Name(w201) -> ("Process_Type"=w199:T22, "Parameter"=w200:string)
                n121 = case shown="Default" w199 {
                  tunnel: w200 -> [_ w205]
                  tunnel: w199 -> [_ w204]
                  frame "None" {
                  }
                  frame Default {
                    n122 = property on="Tab" class="TabCtl (strict)"("Value"=w204) -> ()  [unwired: 2 in, 2 out]
                    n123 = call "AddFuction_EnDisable.vi"("Value"=w204) -> ()  [unwired: 10 in, 1 out]
                    n124 = case shown="\"BinaryMono\"" w204 {
                      tunnel: w205 -> [_ w206 w211 w214 w217 w220 w223 w226 w229]
                      frame "None", Default {
                      }
                      frame "ExtractPlane" {
                        n125 = Variant To Data(type=T20 {"Color Plane"=enum."Blue"} ("ExtractPlanParam"), Variant=w206) -> (data=w207:T20)  [unwired: 1 in, 1 out]
                        n126 = local write "ExtractPlanParam"(w207) -> ()
                      }
                      frame "BinaryMono" {
                        n127 = Variant To Data(type=T4 {"Look For"=enum."Dark Objects", "Threshold"={0.0, 134.0}} ("BinaryMonoParam"), Variant=w211) -> (data=w209:T4)  [unwired: 1 in, 1 out]
                        n128 = local write "BinaryMonoParam"(w209) -> ()
                      }
                      frame "Operators" {
                        n129 = Variant To Data(type=T5 {"Actions"=enum."Multiply", "Select Mode:"=enum."Image", "Color Box"=9221012, "Image Path"=path "\\\\Mac\\Home/Desktop/ssss.png"} ("OperatorsParam"), Variant=w214) -> (data=w213:T5)  [unwired: 1 in, 1 out]
                        n130 = local write "OperatorsParam"(w213) -> ()
                      }
                      frame "GrayMorphology" {
                        n131 = Variant To Data(type=T6 {"Operation"=enum."AutoM", "Structuring Element"=[[1, 1, 1], [1, 1, 1], [1, 1, 1]], "Square/Hexa (Square)"=FALSE, "Number of iterations"=1} ("GrayMorphologyParam"), Variant=w217) -> (data=w215:T6)  [unwired: 1 in, 1 out]
                        n132 = local write "GrayMorphologyParam"(w215) -> ()
                      }
                      frame "Filters" {
                        n133 = Variant To Data(type=T7 {"Kernel"=[[1.0, 1.0, 1.0], [1.0, 1.0, 1.0], [1.0, 1.0, 1.0]], "Kernel Size"=0, "Filter Size X"=0, "Filter Size Y"=0, "Tolerance %"=0, "Divider"=0.0, "FilterFunction"=enum."Smoothing - Low Pass", "Sigma"=0.0, "LThres"=0.0, "HThresh"=0.0, "Windows Size"=0} ("FiltersParam"), Variant=w220) -> (data=w218:T7)  [unwired: 1 in, 1 out]
                        n134 = local write "FiltersParam"(w218) -> ()
                      }
                      frame "Lookup Table" {
                        n135 = Variant To Data(type=T8 {"Function"=enum."Equalizer", "Power Value"=0.0} ("LookupTableParam"), Variant=w223) -> (data=w221:T8)  [unwired: 1 in, 1 out]
                        n136 = local write "LookupTableParam"(w221) -> ()
                      }
                      frame "Particle Filter" {
                        n137 = Variant To Data(type=T9 {"Selection Values"=[{"Measurement Parameter"=0, "Range Lower Value"=0.0, "Range Upper Value"=0.0, "Range"=FALSE, "Measurement Type"=FALSE}], "Keep/Remove Particles (F)"=FALSE, "Reject Border? (F)"=FALSE, "Fill Holes? (F)"=FALSE, "Connectivity 4/8 (8)"=FALSE} ("ParticleFilterParam"), Variant=w226) -> (data=w224:T9)  [unwired: 1 in, 1 out]
                        n138 = local write "ParticleFilterParam"(w224) -> ()
                      }
                      frame "Mask" {
                        n139 = Variant To Data(type=T11 {"Function"=enum."Inside", "ROI List"=0, "ROI"=[], "Creat ROI"=FALSE, "Delete ROI"=FALSE, "Enabled/Disabled"=FALSE, "Color Box"=0, "Last Mouse Position"={"X"=0, "Y"=0}} ("MaskParam"), Variant=w229) -> (data=w227:T11)  [unwired: 1 in, 1 out]
                        n140 = local write "MaskParam"(w227) -> ()
                      }
                    }
                  }
                }
              }
            }
          }
        }
      }
      event "Remove": Value Change {
        n141 = event-data() -> ()  [unwired: 1 in, 1 out]
        n142 = Enqueue Element(queue=w232, element=T17 {"Process_UIActionCmd"=enum."RemoveSteps", "Process_UIParam"=variant, "EventName"=""} ("Process_UIAction"), error in (no error)=w231) -> ()  [unwired: 1 in, 3 out]
      }
      event Value Change {
        n143 = event-data() -> ("CtlRef"=w235:refnum<vi>)  [unwired: 1 in, 5 out]
        n144 = property on="Vision_Image_Show" class="ImageControl"() -> ("ROI"=w233:T26)  [unwired: 2 in, 2 out]
        n145 = property on="Save" class="Bool"() -> ("DisabledEnum"=w238:T14)  [unwired: 2 in, 2 out]
        n146 = case shown="\"Enabled\"" w238 {
          tunnel: w237 -> [w245 _ _]
          tunnel: w236 -> [w246 _ _]
          tunnel: w235 -> [w244 _ w269]
          tunnel: w234 -> [w242 _ _]
          tunnel: w233 -> [w239 _ _]
          frame "Enabled" {
            n147 = Unbundle By Name(w239) -> ("Contours"=w241:T27)
            n148 = Empty Array?(array=w241) -> (empty?=w240:bool)
            n149 = property class="Bool (strict)"(reference=w244, "Value"=FALSE) -> ()  [unwired: 1 in, 2 out]
            n150 = case shown="False" w240 {
              tunnel: w246 -> [w254 _]
              tunnel: w245 -> [w253 _]
              tunnel: w242 -> [w252 _]
              tunnel: w239 -> [w247 _]
              frame False {
                n151 = Unbundle By Name("MaskParam") -> ("Enabled/Disabled"=w249:bool, "Color Box"=w248:u32)
                n152 = call "[FGV]MaskROIDataEntry.vi"("[FGV]MaskROIList_Action"=MaskROIList_Action."Append", "ROIIn"=w247, "error in (no error)"=w254) -> ("error out"=w268:errorcluster)  [unwired: 10 in, 2 out]
                n153 = call "[FGV]MaskROIDataEntry.vi"("[FGV]MaskROIList_Action"=MaskROIList_Action."ReadAll", "error in (no error)"=w268) -> ("ROIArrayOut"=w263:T28, "ROINameOut"=w265:string[])  [unwired: 11 in, 1 out]
                n154 = call "UPdate Mask ROI List.vi"("MaskParam 2"=w252, "Item Names"=w265) -> ("error out"=w255:errorcluster)  [unwired: 9 in]
                n155 = call "[FGV]ProcessDataEntry.vi"("ProcessDataEntry_Action"=ProcessDataEntry_Action."ReallAllSteps") -> ("AllProcessSettingOut"=w260:T12[])  [unwired: 7 in, 3 out]
                n156 = control-ref of="Process Steps"() -> (w258:refnum<vi>)
                n157 = call "Read Mask Paramter.vi"("Type"=Process_Type."Mask", "AllProcessSettingOut"=w260) -> ("data"=w259:T11)  [unwired: 9 in]
                n158 = Bundle By Name(cluster=w259, "Enabled/Disabled"=w249, "ROI"=w263, "Color Box"=w248) -> (w257:T11)
                n159 = call "ProceedProcessSelection.vi"("Error In"=w255, "Selected Param"=w257, "MulticolumnListbox in"=w258) -> ("error out"=w256:errorcluster)  [unwired: 8 in]
                n160 = Enqueue Element(queue=w253, element=T17 {"Process_UIActionCmd"=enum."RunAllSteps", "Process_UIParam"=variant, "EventName"=""}, error in (no error)=w256) -> (error out=w251:errorcluster)  [unwired: 1 in, 2 out]
                n161 = invoke on="Vision_Image_Show" class="ImageControl" method="Clear ROI"(error in=w251) -> ()  [unwired: 2 in, 3 out]
              }
              frame True {
              }
            }
          }
          frame "Disabled", Default {
          }
          frame "Disabled and Grayed Out" {
            n162 = property class="Bool (strict)"(reference=w269, "Value"=FALSE) -> ()  [unwired: 1 in, 2 out]
          }
        }
      }
      event Value Change {
        n163 = event-data() -> ("CtlRef"=w271:refnum<vi>)  [unwired: 1 in, 5 out]
        n164 = property on="Save" class="Bool"() -> ("DisabledEnum"=w273:T14)  [unwired: 2 in, 2 out]
        n165 = case shown="\"Enabled\"" w273 {
          tunnel: w274 -> [w304 _ _]
          tunnel: w272 -> [w303 _ _]
          tunnel: w271 -> [w276 _ w308]
          frame "Enabled" {
            w290 = refnum<vi> refnum  # ListBox
            n166 = property class="Bool (strict)"(reference=w276, "Value"=FALSE) -> ()  [unwired: 1 in, 2 out]
            n167 = property class="Clust (strict)"(reference=w303) -> ("Controls[]"=w293:refnum<vi>[])  [unwired: 1 in, 2 out]
            n168 = Index Array(array=w293, index=1) -> (element=w291:refnum<vi>)
            n169 = To More Specific Class(target class=w290, reference=w291) -> (specific class reference=w289:refnum<vi>)  [unwired: 1 in, 1 out]
            n170 = property class="LstBox"(reference=w289) -> (reference out=w280:refnum<vi>, "Value"=w288:variant)  [unwired: 1 in, 1 out]
            n171 = control-ref of="Process Steps"() -> (w297:refnum<vi>)
            n172 = call "[FGV]ProcessDataEntry.vi"("ProcessDataEntry_Action"=ProcessDataEntry_Action."ReallAllSteps") -> ("AllProcessSettingOut"=w299:T12[])  [unwired: 7 in, 3 out]
            n173 = Variant To Data(type=0, Variant=w288) -> (data=w278:i32, error out=w277:errorcluster)  [unwired: 1 in]
            n174 = call "Read Mask Paramter.vi"("Type"=Process_Type."Mask", "AllProcessSettingOut"=w299) -> ("data"=w298:T11)  [unwired: 9 in]
            n175 = Equal?(x=-1, y=w278) -> (x = y?=w282:bool)
            n176 = case shown="False" w282 {
              tunnel: [w306 _] -> w284
              tunnel: w278 -> [w305 _]
              frame False {
                n177 = invoke on="Vision_Image_Show" class="ImageControl" method="Clear ROI"() -> ()  [unwired: 3 in, 3 out]
                n178 = call "[FGV]MaskROIDataEntry.vi"("[FGV]MaskROIList_Action"=MaskROIList_Action."DeleteIndex", "Replace index"=w305) -> ("error out"=w306:errorcluster)  [unwired: 11 in, 2 out]
              }
              frame True {
              }
            }
            n179 = call "[FGV]MaskROIDataEntry.vi"("[FGV]MaskROIList_Action"=MaskROIList_Action."ReadAll", "error in (no error)"=w284) -> ("ROIArrayOut"=w283:T28, "ROINameOut"=w281:string[])  [unwired: 11 in, 1 out]
            n180 = call "UPdate Mask ROI List.vi"("MaskParam 2"=w303, "Item Names"=w281) -> ("error out"=w294:errorcluster)  [unwired: 9 in]
            n181 = Bundle By Name(cluster=w298, "ROI"=w283) -> (w296:T11)
            n182 = property class="LstBox"(reference=w280, error in=w277, "Value"=-1) -> ()  [unwired: 2 out]
            n183 = call "ProceedProcessSelection.vi"("Error In"=w294, "Selected Param"=w296, "MulticolumnListbox in"=w297) -> ("error out"=w295:errorcluster)  [unwired: 8 in]
            n184 = Enqueue Element(queue=w304, element=T17 {"Process_UIActionCmd"=enum."RunAllSteps", "Process_UIParam"=variant, "EventName"=""}, error in (no error)=w295) -> ()  [unwired: 1 in, 3 out]
          }
          frame "Disabled", Default {
          }
          frame "Disabled and Grayed Out" {
            n185 = property class="Bool (strict)"(reference=w308, "Value"=FALSE) -> ()  [unwired: 1 in, 2 out]
          }
        }
      }
      event Value Change {
        n186 = event-data() -> ("NewVal"=w313:i32)  [unwired: 1 in, 5 out]
        n187 = property on="Save" class="Bool"() -> ("DisabledEnum"=w314:T14)  [unwired: 2 in, 2 out]
        n188 = case shown="\"Enabled\"" w314 {
          tunnel: w313 -> [w317 _ _]
          tunnel: w312 -> [_ _ _]
          tunnel: w311 -> [w319 _ _]
          tunnel: w310 -> [_ _ _]
          frame "Enabled" {
            n189 = call "[FGV]MaskROIDataEntry.vi"("[FGV]MaskROIList_Action"=MaskROIList_Action."ReadAll", "error in (no error)"=w319) -> ("ROIArrayOut"=w318:T28)  [unwired: 11 in, 2 out]
            n190 = Index Array(array=w318, index=w317) -> (element=w316:T26)
            n191 = property on="Vision_Image_Show" class="ImageControl"("ROI"=w316) -> ()  [unwired: 2 in, 2 out]
          }
          frame "Disabled", Default {
          }
          frame "Disabled and Grayed Out" {
          }
        }
      }
      event Value Change {
        n192 = event-data() -> ("NewVal"=w323:enum16{"Inside", "Outside"})  [unwired: 1 in, 5 out]
        n193 = property on="Save" class="Bool"() -> ("DisabledEnum"=w324:T14)  [unwired: 2 in, 2 out]
        n194 = case shown="\"Enabled\"" w324 {
          tunnel: w323 -> [w328 _ _]
          tunnel: w322 -> [w332 _ _]
          tunnel: w321 -> [w331 _ _]
          tunnel: w320 -> [w330 _ _]
          frame "Enabled" {
            w329 = T17 {"Process_UIActionCmd"=enum."RunAllSteps", "Process_UIParam"=variant, "EventName"=""}  # element
            n195 = local read "MaskParam"() -> (w325:T11)
            n196 = Unbundle By Name(w325) -> ("Color Box"=w327:u32, "Enabled/Disabled"=w326:bool)
            n197 = call "[FGV]MaskROIDataEntry.vi"("[FGV]MaskROIList_Action"=MaskROIList_Action."ReadAll") -> ("ROIArrayOut"=w341:T28, "ROINameOut"=w343:string[])  [unwired: 12 in, 1 out]
            n198 = control-ref of="Process Steps"() -> (w337:refnum<vi>)
            n199 = call "[FGV]ProcessDataEntry.vi"("ProcessDataEntry_Action"=ProcessDataEntry_Action."ReallAllSteps") -> ("AllProcessSettingOut"=w339:T12[])  [unwired: 7 in, 3 out]
            n200 = call "UPdate Mask ROI List.vi"("error in (no error)"=w330, "MaskParam 2"=w331, "Item Names"=w343) -> ("error out"=w334:errorcluster)  [unwired: 8 in]
            n201 = call "Read Mask Paramter.vi"("Type"=Process_Type."Mask", "AllProcessSettingOut"=w339) -> ("data"=w338:T11)  [unwired: 9 in]
            n202 = Bundle By Name(cluster=w338, "ROI"=w341, "Function"=w328, "Color Box"=w327, "Enabled/Disabled"=w326) -> (w336:T11)
            n203 = call "ProceedProcessSelection.vi"("Error In"=w334, "Selected Param"=w336, "MulticolumnListbox in"=w337) -> ("error out"=w335:errorcluster)  [unwired: 8 in]
            n204 = Enqueue Element(queue=w332, element=w329, error in (no error)=w335) -> (error out=w333:errorcluster)  [unwired: 1 in, 2 out]
            n205 = invoke on="Vision_Image_Show" class="ImageControl" method="Clear ROI"(error in=w333) -> ()  [unwired: 2 in, 3 out]
          }
          frame "Disabled", Default {
          }
          frame "Disabled and Grayed Out" {
          }
        }
      }
      event Value Change {
        n206 = event-data() -> ("NewVal"=w345:u32)  [unwired: 1 in, 5 out]
        n207 = property on="Save" class="Bool"() -> ("DisabledEnum"=w350:T14)  [unwired: 2 in, 2 out]
        n208 = case shown="\"Enabled\"" w350 {
          tunnel: w349 -> [w356 _ _]
          tunnel: w348 -> [w355 _ _]
          tunnel: w347 -> [w354 _ _]
          tunnel: w346 -> [_ _ _]
          tunnel: w345 -> [w353 _ _]
          frame "Enabled" {
            n209 = Greater?(x=w353, y=u32 255) -> (0:w351:bool)
            n210 = case shown="False" w351 {
              tunnel: w356 -> [w363 _]
              tunnel: w355 -> [w362 _]
              tunnel: w354 -> [w361 _]
              tunnel: w353 -> [w357 _]
              frame False {
                w364 = T17 {"Process_UIActionCmd"=enum."RunAllSteps", "Process_UIParam"=variant, "EventName"=""}  # element
                n211 = local read "MaskParam"() -> (w359:T11)
                n212 = Unbundle By Name(w359) -> ("Enabled/Disabled"=w358:bool)
                n213 = call "[FGV]MaskROIDataEntry.vi"("[FGV]MaskROIList_Action"=MaskROIList_Action."ReadAll") -> ("ROIArrayOut"=w372:T28, "ROINameOut"=w374:string[])  [unwired: 12 in, 1 out]
                n214 = call "UPdate Mask ROI List.vi"("error in (no error)"=w363, "MaskParam 2"=w361, "Item Names"=w374) -> ("error out"=w366:errorcluster)  [unwired: 8 in]
                n215 = control-ref of="Process Steps"() -> (w368:refnum<vi>)
                n216 = call "[FGV]ProcessDataEntry.vi"("ProcessDataEntry_Action"=ProcessDataEntry_Action."ReallAllSteps") -> ("AllProcessSettingOut"=w370:T12[])  [unwired: 7 in, 3 out]
                n217 = call "Read Mask Paramter.vi"("Type"=Process_Type."Mask", "AllProcessSettingOut"=w370) -> ("data"=w369:T11)  [unwired: 9 in]
                n218 = Bundle By Name(cluster=w369, "ROI"=w372, "Color Box"=w357, "Enabled/Disabled"=w358) -> (w360:T11)
                n219 = call "ProceedProcessSelection.vi"("Error In"=w366, "Selected Param"=w360, "MulticolumnListbox in"=w368) -> ("error out"=w367:errorcluster)  [unwired: 8 in]
                n220 = Enqueue Element(queue=w362, element=w364, error in (no error)=w367) -> (error out=w365:errorcluster)  [unwired: 1 in, 2 out]
                n221 = invoke on="Vision_Image_Show" class="ImageControl" method="Clear ROI"(error in=w365) -> ()  [unwired: 2 in, 3 out]
              }
              frame True {
              }
            }
          }
          frame "Disabled", Default {
          }
          frame "Disabled and Grayed Out" {
          }
        }
      }
      event "Vision_Image_Show": Mouse Up {
        n222 = event-data() -> ("CtlRef"=w377:refnum<vi>)  [unwired: 1 in]
        n223 = property on="Process Steps" class="MCListbox (strict)"() -> ("ItemNames"=w380:string[][], "Value"=w381:i32)  [unwired: 2 in, 2 out]
        n224 = property on="Tab" class="TabCtl (strict)"() -> ("Value"=w386:T2)  [unwired: 2 in, 2 out]
        n225 = property class="ImageControl"(reference=w377) -> ("Last Mouse Position"=w376:cluster{"X":i32, "Y":i32})  [unwired: 1 in, 2 out]
        n226 = Index Array(array=w380, index (row)=w381, index (col)=0 ("disabled index (col)")) -> (element=w383:string)
        n227 = Equal?(x=w383, y="Mask") -> (x = y?=w379:bool)
        n228 = case shown="\"Mask\"" w386 {
          tunnel: w385 -> [_ _ _ _ _ _ _ _ w390]
          tunnel: w379 -> [_ _ _ _ _ _ _ _ w389]
          tunnel: w378 -> [_ _ _ _ _ _ _ _ w388]
          tunnel: w376 -> [_ _ _ _ _ _ _ _ w387]
          frame "None", Default {
          }
          frame "ExtractPlane" {
          }
          frame "ExtractPlane" {
          }
          frame "Operators" {
          }
          frame "GrayMorphology" {
          }
          frame "Filters" {
          }
          frame "Lookup Table" {
          }
          frame "Particle Filter" {
          }
          frame "Mask" {
            n229 = case shown="True" w389 {
              tunnel: w390 -> [_ w421]
              tunnel: w388 -> [_ w405]
              tunnel: w387 -> [_ w394]
              frame False {
              }
              frame True {
                w410 = refnum<vi> refnum  # ListBox
                n230 = property class="Clust (strict)"(reference=w405) -> ("Controls[]"=w413:refnum<vi>[])  [unwired: 1 in, 2 out]
                n231 = property on="Vision_Image_Show" class="ImageControl"() -> ("ROI"=w406:T26)  [unwired: 2 in, 2 out]
                n232 = local read "MaskParam"() -> (w393:T11)
                n233 = Unbundle By Name(w393) -> ("Enabled/Disabled"=w392:bool, "Color Box"=w391:u32)
                n234 = Index Array(array=w413, index=1) -> (element=w411:refnum<vi>)
                n235 = To More Specific Class(target class=w410, reference=w411) -> (specific class reference=w409:refnum<vi>)  [unwired: 1 in, 1 out]
                n236 = property class="LstBox"(reference=w409) -> (reference out=w398:refnum<vi>, "Value"=w408:variant)  [unwired: 1 in, 1 out]
                n237 = control-ref of="Process Steps"() -> (w417:refnum<vi>)
                n238 = call "[FGV]ProcessDataEntry.vi"("ProcessDataEntry_Action"=ProcessDataEntry_Action."ReallAllSteps") -> ("AllProcessSettingOut"=w419:T12[])  [unwired: 7 in, 3 out]
                n239 = Variant To Data(type=0, Variant=w408) -> (data=w396:i32, error out=w395:errorcluster)  [unwired: 1 in]
                n240 = call "Read Mask Paramter.vi"("Type"=Process_Type."Mask", "AllProcessSettingOut"=w419) -> ("data"=w418:T11)  [unwired: 9 in]
                n241 = Equal?(x=-1, y=w396) -> (x = y?=w400:bool)
                n242 = case shown="False" w400 {
                  tunnel: w406 -> [w427 _]
                  tunnel: [w425 _] -> w402
                  tunnel: w396 -> [w424 _]
                  frame False {
                    n243 = invoke on="Vision_Image_Show" class="ImageControl" method="Clear ROI"() -> ()  [unwired: 3 in, 3 out]
                    n244 = call "[FGV]MaskROIDataEntry.vi"("[FGV]MaskROIList_Action"=MaskROIList_Action."Replace", "ROIIn"=w427, "Replace index"=w424) -> ("error out"=w425:errorcluster)  [unwired: 10 in, 2 out]
                  }
                  frame True {
                  }
                }
                n245 = call "[FGV]MaskROIDataEntry.vi"("[FGV]MaskROIList_Action"=MaskROIList_Action."ReadAll", "error in (no error)"=w402) -> ("ROIArrayOut"=w401:T28, "ROINameOut"=w399:string[])  [unwired: 11 in, 1 out]
                n246 = call "UPdate Mask ROI List.vi"("MaskParam 2"=w405, "Item Names"=w399) -> ("error out"=w414:errorcluster)  [unwired: 9 in]
                n247 = Bundle By Name(cluster=w418, "Enabled/Disabled"=w392, "Color Box"=w391, "Last Mouse Position"=w394, "ROI"=w401) -> (w416:T11)
                n248 = property class="LstBox"(reference=w398, error in=w395, "Value"=-1) -> ()  [unwired: 2 out]
                n249 = call "ProceedProcessSelection.vi"("Error In"=w414, "Selected Param"=w416, "MulticolumnListbox in"=w417) -> ("error out"=w415:errorcluster)  [unwired: 8 in]
                n250 = Enqueue Element(queue=w421, element=T17 {"Process_UIActionCmd"=enum."RunAllSteps", "Process_UIParam"=variant, "EventName"=""}, error in (no error)=w415) -> ()  [unwired: 1 in, 3 out]
              }
            }
          }
        }
      }
    }
    "Cancel?" <- w68
  }
  n251 = while {
    tunnel: w23 -> [w457]
    tunnel: w17 -> [w456]
    shift-right: [w439] -> w24
    shift-left: w15 -> [w453]
    tunnel: [w433] -> w25
    shift-right: [w438] -> w13
    shift-left: w12 -> [w448]
    tunnel: [w440] -> w8
    shift-right: [w431] -> _
    shift-left: _ -> [w430]
    shift-right: [w429] -> _
    shift-left: w3 -> [w428]
    stop <- w452 stop-if-true
    n252 = Dequeue Element(queue=w457, error in (no error)=w456) -> (queue out=w434:refnum<queue>, element=w455:T17, error out=w445:errorcluster)  [unwired: 1 in, 1 out]
    n253 = call "[FGV]ProcessDataEntry.vi"("ProcessDataEntry_Action"=ProcessDataEntry_Action."ReallAllSteps", "Error In"=w445) -> ("Error Out"=w436:errorcluster, "AllProcessSettingOut"=w446:T12[])  [unwired: 6 in, 2 out]
    n254 = Unbundle(w455) -> ("Process_UIActionCmd"=w454:T30, "Process_UIParam"=w451:variant, "EventName"=w449:string)
    n255 = case shown="\"RunAllSteps\"" w454 {
      tunnel: w446 -> [_ w496 w530 w575 w629]
      tunnel: w453 -> [w468 w479 w536 w585 w628]
      tunnel: [w461 w485 w531 w591 w629] -> w432
      tunnel: [w468 w484 w544 w584 w628] -> w439
      tunnel: [_ _ _ _ TRUE] -> w452
      tunnel: w451 -> [_ w494 _ _ _]
      tunnel: w449 -> [_ w489 _ _ _]
      tunnel: w448 -> [w473 w488 w537 w594 w626]
      tunnel: [w473 w482 w533 w586 w626] -> w438
      tunnel: [w463 w487 w527 w581 w625] -> w437
      tunnel: w436 -> [w470 _ w540 w592 w625]
      tunnel: w434 -> [w469 w481 w538 w576 w624]
      tunnel: [w469 w481 w538 w576 w624] -> w433
      tunnel: [T1 refnum ("ExtractImageOut") w478 w526 w573 w623] -> w431
      tunnel: w430 -> [_ w477 w525 w573 w623]
      tunnel: w428 -> [w466 w476 w524 w572 w622]
      tunnel: [w465 w475 w523 w571 w622] -> w429
      frame "Init", Default {
        n256 = call "[FGV] Control_Eanble_Disable.vi"("Control_EnDisable_Action"=Control_EnDisable_Action."Enable All", "Error In"=w470) -> ("Error Out"=w471:errorcluster)  [unwired: 8 in, 1 out]
        n257 = call "[FGV]ProcessDataEntry.vi"("ProcessDataEntry_Action"=ProcessDataEntry_Action."ReallAllSteps", "Error In"=w471) -> ("Error Out"=w464:errorcluster, "AllProcessSettingOut"=w462:T12[])  [unwired: 6 in, 2 out]
        n258 = call "UPdate MaskROIDataEntry.vi"("AllProcessSettingIn"=w462, "error in (no error)"=w464) -> ("AllProcessSettingOut"=w461:T12[], "ROIName"=w460:string[], "Enabled/Disabled"=w459:bool, "Color Box"=w458:u32, "error out"=w463:errorcluster)  [unwired: 9 in]
        n259 = call "UPdate Mask Paramter.vi"("Color Box"=w458, "Enabled/Disabled"=w459, "ROIName"=w460, "Cluster in"=w466) -> ("Cluster out"=w465:refnum<vi>)  [unwired: 7 in]
      }
      frame "SingleStep" {
        n260 = Variant To Data(type=cluster{"Value":T29, "Value":variant} {"Value"=enum."BinaryMono", "Value"=variant} ("output cluster"), Variant=w494) -> (data=w493:cluster{"Value":T29, "Value":variant})  [unwired: 1 in, 1 out]
        n261 = Unbundle(w493) -> ("Value"=w490:T29, "Value"=w491:variant)
        n262 = call "SetImageDisplayType.vi"("Value"=w490) -> ("Palette:Palette Type"=w492:u32)  [unwired: 9 in, 1 out]
        n263 = property on="Vision_Image_Show" class="ImageControl"("Palette Type"=w492) -> ()  [unwired: 2 in, 2 out]
        n264 = call "Execute_Single_Process.vi"("Tab Control"=w490, "MaskParam 2"=w476, "Parameter"=w491, "ImageIn"=w479, "ExtractImageControl"=w477, "OperatorImage"=w488) -> ("MaskParam 4"=w475:refnum<vi>, "ProcessSettingOut"=w498:T12, "ExtractImage"=w478:T1, "Image Out"=w499:T1, "OperatorImageOut"=w480:T1, "error out"=w497:errorcluster)  [unwired: 4 in]
        n265 = case shown="Error" w497 {
          selector: w497 -> [w500 w515]
          tunnel: w499 -> [w502 w521]
          tunnel: w496 -> [w505 w522]
          tunnel: w498 -> [w506 _]
          tunnel: [w504 w522] -> w485
          tunnel: [w502 w521] -> w484
          tunnel: w480 -> [w501 w520]
          tunnel: w489 -> [w503 _]
          tunnel: [w501 w520] -> w482
          tunnel: [w500 w516] -> w483
          frame No Error {
            n266 = case shown="\"False\", Default" w503 {
              tunnel: w506 -> [w511 w513]
              tunnel: w505 -> [w510 w514]
              tunnel: [w509 w512] -> w504
              frame "False", Default {
                n267 = Array Size(array=w510) -> (size(s)=w508:i32)
                n268 = Decrement(x=w508) -> (x-1=w507:i32)
                n269 = Replace Array Subset(array=w510, new element=w511, index=w507) -> (w509:T12[])
              }
              frame "Add" {
                n270 = Build Array (concatenate)(w514, w513) -> (w512:T12[])
              }
            }
          }
          frame Error {
            n271 = call "ProcessErrorHandle.vi"("error in (no error)"=w515) -> ()  [unwired: 10 in, 1 out]
            n272 = call "[FGV] Control_Eanble_Disable.vi"("Control_EnDisable_Action"=Control_EnDisable_Action."Select Mode") -> ("Error Out"=w518:errorcluster)  [unwired: 9 in, 1 out]
            n273 = call "[FGV] Control_Eanble_Disable.vi"("Control_EnDisable_Action"=Control_EnDisable_Action."AllPageEnable", "Error In"=w518) -> ("Error Out"=w516:errorcluster)  [unwired: 8 in, 1 out]
          }
        }
        n274 = control-ref of="Process Steps"() -> (w486:refnum<vi>)
        n275 = call "PrcoessStepFocus.vi"("Error In"=w483, "AllProcessSettingOut"=w485, "MulticolumnListbox in"=w486) -> ("Error Out"=w487:errorcluster)  [unwired: 8 in]
      }
      frame "RunAllSteps" {
        # "Define Error Code"
        n276 = local read "Vision_Image_In"() -> (w543:T1)
        n277 = call "CreateNewImage.vi"("Error In"=w540, "Display Image In"=w536, "Image Name"="RunAllStepTemp1", "Original Image"=w543) -> ("Error Out"=w539:errorcluster, "Orignal Image Temp Out"=w541:T1)  [unwired: 5 in, 1 out]
        n278 = call "Execute_All_Process.vi"("OperatorImage In"=w537, "MaskParam 2"=w524, "error in (no error)"=w539, "ImageIn"=w541, "ExtractImageIn"=w525, "ProcessSettingIn"=w530) -> ("error out"=w534:errorcluster, "Image Out"=w535:T1, "ExtractImageOut"=w526:T1, "Palette Type"=w545:u32, "OperatorImage Out"=w532:T1, "MaskParam 3"=w523:refnum<vi>)
        n279 = case shown="Error" w534 {
          selector: w534 -> [w548 w570]
          tunnel: w545 -> [w546 _]
          tunnel: [w549 w560] -> w544
          tunnel: w536 -> [w551 w557]
          tunnel: w535 -> [w550 w554]
          tunnel: [w553 w555] -> w533
          tunnel: w532 -> [w553 w556]
          tunnel: [w552 w558] -> w531
          tunnel: w530 -> [w552 _]
          tunnel: [w547 w562] -> w528
          tunnel: [w546 w559] -> w529
          frame No Error {
            n280 = call "CopyClearTempImage.vi"("error in (no error)"=w548, "Display Image In"=w551, "TempImageRefIn"=w550) -> ("error out"=w547:errorcluster, "DisplayImageOut"=w549:T1)  [unwired: 7 in]
          }
          frame Error {
            n281 = local read "Vision_Image_In"() -> (w566:T1)
            n282 = call "ProcessErrorHandle.vi"("error in (no error)"=w570) -> ("error out (no error)"=w567:errorcluster)  [unwired: 10 in]
            n283 = call "Imaq Dispose"("Image"=w554) -> ()  [unwired: 5 in, 1 out]
            n284 = call "[FGV]ProcessDataEntry.vi"("ProcessDataEntry_Action"=ProcessDataEntry_Action."ReallAllSteps") -> ("OldAllProcessSetting Out"=w558:T12[])  [unwired: 7 in, 3 out]
            n285 = call "CreateNewImage.vi"("Error In"=w567, "Image Name"="RunAllStepTemp2", "Original Image"=w566) -> ("Error Out"=w569:errorcluster, "Orignal Image Temp Out"=w568:T1)  [unwired: 6 in, 1 out]
            n286 = call "Execute_All_Process.vi"("OperatorImage In"=w556, "error in (no error)"=w569, "ImageIn"=w568, "ProcessSettingIn"=w558) -> ("error out"=w563:errorcluster, "Image Out"=w561:T1, "Palette Type"=w559:u32, "OperatorImage Out"=w555:T1)  [unwired: 2 in, 2 out]
            n287 = call "CopyClearTempImage.vi"("error in (no error)"=w563, "Display Image In"=w557, "TempImageRefIn"=w561) -> ("error out"=w562:errorcluster, "DisplayImageOut"=w560:T1)  [unwired: 7 in]
          }
        }
        n288 = property on="Vision_Image_Show" class="ImageControl"(error in=w528, "Palette Type"=w529) -> (error out=w527:errorcluster)  [unwired: 1 in, 1 out]
      }
      frame "RemoveSteps" {
        n289 = local read "Vision_Image_In"() -> (w583:T1)
        n290 = property on="Process Steps" class="MCListbox (strict)"() -> ("Value"=w596:i32)  [unwired: 2 in, 2 out]
        n291 = for {
          N: 2 -> [_]
          tunnel: w583 -> [w600]
          tunnel: w585 -> [w597]
          tunnel: [w601] -> w579 mode=indexing
          tunnel: [w597] -> w574
          i -> [w599]
          n292 = Number To Decimal String(number=w599) -> (decimal integer string=w598:string)  [unwired: 1 in]
          n293 = call "CreateNewImage.vi"("Display Image In"=w597, "Image Name"=w598, "Original Image"=w600) -> ("Orignal Image Temp Out"=w601:T1)  [unwired: 6 in, 2 out]
        }
        n294 = Delete From Array(array=w575, index=w596) -> (array with subset deleted=w590:T12[])  [unwired: 1 in, 1 out]
        n295 = Index Array(array=w579) -> (element #1=w578:T1, element #2=w577:T1)  [unwired: 2 in]
        n296 = call "Execute_All_Process.vi"("OperatorImage In"=w594, "MaskParam 2"=w572, "error in (no error)"=w592, "ImageIn"=w578, "ProcessSettingIn"=w590) -> ("error out"=w593:errorcluster, "Image Out"=w589:T1, "Palette Type"=w595:u32, "OperatorImage Out"=w587:T1, "MaskParam 3"=w571:refnum<vi>)  [unwired: 1 in, 1 out]
        n297 = case shown="No Error" w593 {
          selector: w593 -> [w607 w621]
          tunnel: w595 -> [w608 _]
          tunnel: [w609 w619] -> w591
          tunnel: w575 -> [_ w619]
          tunnel: w590 -> [w609 _]
          tunnel: [w606 w614] -> w582
          tunnel: w589 -> [w604 w611]
          tunnel: w574 -> [w602 w612]
          tunnel: [w605 w615] -> w584
          tunnel: w577 -> [_ w620]
          tunnel: [w608 w618] -> w588
          tunnel: w587 -> [w603 w617]
          tunnel: [w603 w616] -> w586
          frame No Error {
            n298 = call "CopyClearTempImage.vi"("error in (no error)"=w607, "Display Image In"=w602, "TempImageRefIn"=w604) -> ("error out"=w606:errorcluster, "DisplayImageOut"=w605:T1)  [unwired: 7 in]
          }
          frame Error {
            n299 = call "Imaq Dispose"("Image"=w611) -> ()  [unwired: 5 in, 1 out]
            n300 = call "Execute_All_Process.vi"("OperatorImage In"=w617, "ImageIn"=w620, "ProcessSettingIn"=w619) -> ("error out"=w610:errorcluster, "Image Out"=w613:T1, "Palette Type"=w618:u32, "OperatorImage Out"=w616:T1)  [unwired: 3 in, 2 out]
            n301 = call "ProcessErrorHandle.vi"("error in (no error)"=w621) -> ()  [unwired: 10 in, 1 out]
            n302 = call "CopyClearTempImage.vi"("error in (no error)"=w610, "Display Image In"=w612, "TempImageRefIn"=w613) -> ("error out"=w614:errorcluster, "DisplayImageOut"=w615:T1)  [unwired: 7 in]
          }
        }
        n303 = property on="Vision_Image_Show" class="ImageControl"(error in=w582, "Palette Type"=w588) -> (error out=w581:errorcluster)  [unwired: 1 in, 1 out]
      }
      frame "Exist" {
      }
    }
    n304 = call "[FGV]ProcessDataEntry.vi"("ProcessDataEntry_Action"=ProcessDataEntry_Action."UpdateSteps", "Error In"=w437, "OldAllProcessSetting In"=w432, "AllProcessSetting In"=w432) -> ("Error Out"=w442:errorcluster)  [unwired: 4 in, 3 out]
    n305 = control-ref of="Process Steps"() -> (w435:refnum<vi>)
    n306 = local write "Operators_Image"(w438) -> ()
    n307 = local write "Vision_Image_Show"(w439) -> ()
    n308 = call "[FGV]ProcessDataEntry.vi"("ProcessDataEntry_Action"=ProcessDataEntry_Action."ReallAllSteps", "Error In"=w442) -> ("Error Out"=w444:errorcluster, "AllProcessSettingOut"=w443:T12[])  [unwired: 6 in, 2 out]
    n309 = call "Show_Process_Steps.vi"("error in (no error)"=w444, "ProcessSettingIn"=w443, "ProcessSteps"=w435) -> ("error out"=w440:errorcluster)  [unwired: 8 in]
  }
  n310 = Release Queue(queue=w25) -> ()  [unwired: 2 in, 3 out]
  n311 = call "[FGV]ProcessDataEntry.vi"("ProcessDataEntry_Action"=ProcessDataEntry_Action."ReallAllSteps", "Error In"=w8) -> ("AllProcessSettingOut"=→"ProcessSettingOut":T12[])  [unwired: 6 in, 3 out]
  n312 = call "Imaq Dispose"("Image"=w24) -> ()  [unwired: 5 in, 1 out]
  n313 = call "Imaq Dispose"("Image"=w13) -> ()  [unwired: 5 in, 1 out]
